vi "ma_SML Averaged FFT Power Spectrum.vi"(6 "reset averaging?":bool, 8 "error in (no error)":errorcluster, 9 "averaging parameters":T1={"averaging type"=enum."no averaging", "averaging settings"={"weighting type"=enum."linear", "weighting settings"={"size"=10.0, "linear weighting mode"=enum."moving average"}}}, 10 "spectral info in":T5 {"window" items=["Rectangle"=0, "Hanning"=1, "Hamming"=2, "Blackman-Harris"=3, "Exact Blackman"=4, "Blackman"=5, "Flat Top"=6, "4 Term B-Harris "=7, "7 Term B-Harris"=8, "Low Sidelobe"=9, "Blackman Nuttall"=11, "Triangle"=30, "Bartlett-Hanning"=31, "Bohman"=32, "Parzen"=33, "Welch"=34, "Kaiser"=60, "Dolph-Chebyshev"=61, "Gaussian"=62]}, 11 "FFT spectrum":T4 {"spectrum" format="%.2f"; "df" format="%.2f"; "f0" format="%.2f"}) -> (0 "error out":errorcluster, 1 "data ready?":bool, 2 "spectral info out":T5 {"window" items=["Rectangle"=0, "Hanning"=1, "Hamming"=2, "Blackman-Harris"=3, "Exact Blackman"=4, "Blackman"=5, "Flat Top"=6, "4 Term B-Harris "=7, "7 Term B-Harris"=8, "Low Sidelobe"=9, "Blackman Nuttall"=11, "Triangle"=30, "Bartlett-Hanning"=31, "Bohman"=32, "Parzen"=33, "Welch"=34, "Kaiser"=60, "Dolph-Chebyshev"=61, "Gaussian"=62]}, 3 "avg power spectrum":T3 {"spectrum" format="%.2f"; "df" format="%.2f"; "f0" format="%.2f"}, 4 "averages sofar":dbl)   [LabVIEW 2020, in "NI_MAPro.lvlib"]
uses:
  NI_MAPro.lvlib
  ma_sml_Spectral Info.ctl
  ma_sml_Spectrum Cluster (complex).ctl
  ma_sml_Spectrum Cluster (real).ctl
  ma_sml_Averaging Parameters.ctl
  ma_sml_Averaging Settings.ctl
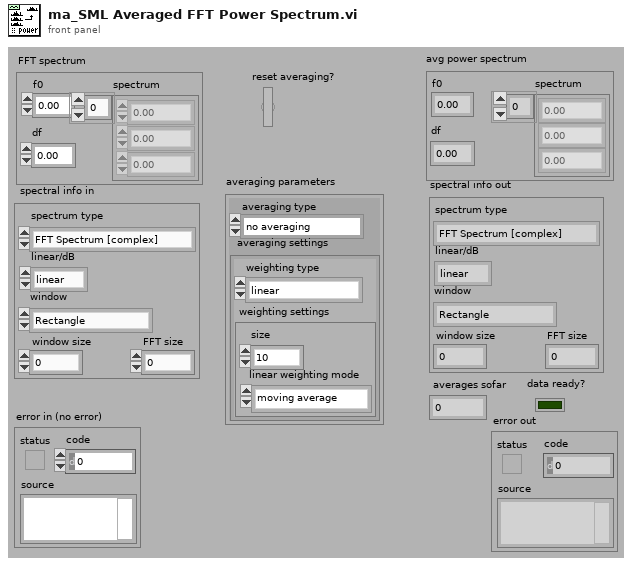
[diagram p1: front panel]
types:
  T1 = typedef "NI_MAPro.lvlib/ma_sml_Averaging Parameters.ctl" = cluster{"averaging type":enum16{"no averaging", "vector averaging", "RMS averaging", "peak hold"}, "averaging settings":T2}
  T2 = typedef "NI_MAPro.lvlib/ma_sml_Averaging Settings.ctl" = cluster{"weighting type":enum16{"linear", "exponential"}, "weighting settings":cluster{"size":dbl, "linear weighting mode":enum16{"one shot", "auto restart one shot", "moving average", "continuous"}}}
  T3 = typedef "NI_MAPro.lvlib/ma_sml_Spectrum Cluster (real).ctl" = cluster{"f0":dbl, "df":dbl, "spectrum":dbl[]}
  T4 = typedef "NI_MAPro.lvlib/ma_sml_Spectrum Cluster (complex).ctl" = cluster{"f0":dbl, "df":dbl, "spectrum":cdb[]}
  T5 = typedef "NI_MAPro.lvlib/ma_sml_Spectral Info.ctl" = cluster{"spectrum type":enum16{"FFT Spectrum [complex]", "Amplitude [Magnitude]", "Power [Magnitude^2]", "Cross Spectrum [complex]", "Frequency Response [Complex]"}, "linear/dB":enum16{"linear", "dB"}, "window":u16, "window size":i32, "FFT size":i32}
  T6 = enum16{"FFT Spectrum [complex]", "Amplitude [Magnitude]", "Power [Magnitude^2]", "Cross Spectrum [complex]", "Frequency Response [Complex]"}
  T7 = enum16{"no averaging", "vector averaging", "RMS averaging", "peak hold"}
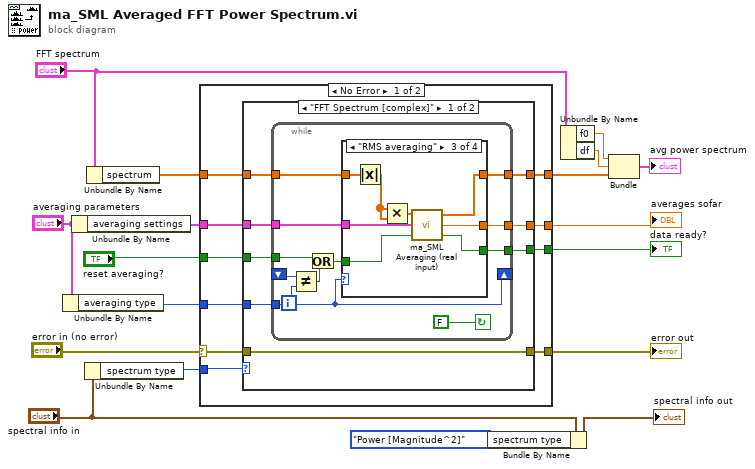
[diagram p0: block diagram]
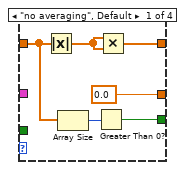
[diagram p2: hidden frame]
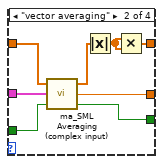
[diagram p3: hidden frame]
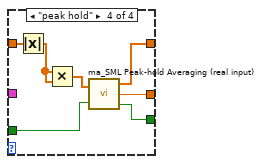
[diagram p4: hidden frame]
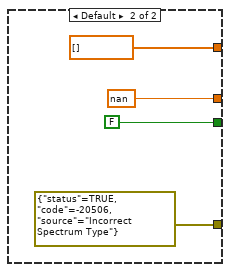
[diagram p5: hidden frame]
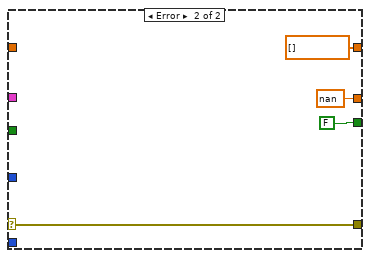
[diagram p6: hidden frame]
diagram:
  n1 = Unbundle By Name("averaging parameters") -> ("averaging type"=w7:T7)
  n2 = Unbundle By Name("averaging parameters") -> ("averaging settings"=w9:T2)
  n3 = Unbundle By Name("spectral info in") -> ("spectrum type"=w12:T6)
  n4 = Unbundle By Name("FFT spectrum") -> ("spectrum"=w16:cdb[])
  n5 = case shown="No Error" "error in (no error)" {
    selector: "error in (no error)" -> [w19 w81]
    tunnel: [w22 FALSE ("Data Ready")] -> w18
    tunnel: [w28 nan ("Averaged So-far")] -> w17
    tunnel: [w27 dbl[] [] ("y")] -> w14
    tunnel: w7 -> [w26 _]
    tunnel: w9 -> [w25 _]
    tunnel: "reset averaging?" -> [w24 _]
    tunnel: w16 -> [w23 _]
    tunnel: [w20 w81] -> w3
    tunnel: w12 -> [w21 _]
    frame No Error {
      n6 = case shown="\"FFT Spectrum [complex]\"" w21 {
        tunnel: [w36 nan ("Averaged So-far")] -> w28
        tunnel: [w35 dbl[] [] ("y")] -> w27
        tunnel: w26 -> [w34 _]
        tunnel: w25 -> [w33 _]
        tunnel: w24 -> [w32 _]
        tunnel: w23 -> [w29 _]
        tunnel: [w30 FALSE] -> w22
        tunnel: w19 -> [w31 _]
        tunnel: [w31 errorcluster {"status"=TRUE, "code"=-20506, "source"="Incorrect Spectrum Type"} ("error in (no error)")] -> w20
        frame "FFT Spectrum [complex]" {
          n7 = while {
            tunnel: w33 -> [w40]
            shift-left: _ -> [w38]
            shift-right: [w37] -> _
            tunnel: w34 -> [w37]
            tunnel: w32 -> [w42]
            tunnel: [w44] -> w36
            tunnel: [w45] -> w30
            tunnel: [w46] -> w35
            tunnel: w29 -> [w47]
            stop <- FALSE continue-if-true
            n8 = Not Equal?(x=w38, y=w37) -> (x != y?=w41:bool)
            n9 = Or(x=w42, y=w41) -> (x .or. y?=w43:bool)
            n10 = case shown="\"RMS averaging\"" w37 {
              tunnel: [w52 w56 w63 w74] -> w46
              tunnel: w47 -> [w50 w61 w69 w75]
              tunnel: [w48 w58 w65 w70] -> w45
              tunnel: [0.0 ("Averaged So-far") w59 w66 w73] -> w44
              tunnel: w43 -> [_ w60 w64 w76]
              tunnel: w40 -> [_ w54 w62 _]
              frame "no averaging", Default {
                n11 = Absolute Value(x=w50) -> (abs(x)=w51:dbl[])
                n12 = Array Size(array=w50) -> (size(s)=w49:i32)
                n13 = Greater Than 0?(x=w49) -> (x > 0?=w48:bool)
                n14 = Multiply(x=w51, y=w51) -> (x*y=w52:dbl[])
              }
              frame "vector averaging" {
                n15 = call "ma_SML Averaging (complex input).vi"("reset?"=w60, "averaging settings"=w54, "x"=w61) -> ("data ready?"=w58:bool, "averaged sofar"=w59:dbl, "y"=w57:cdb[])
                n16 = Absolute Value(x=w57) -> (abs(x)=w55:dbl[])
                n17 = Multiply(x=w55, y=w55) -> (x*y=w56:dbl[])
              }
              frame "RMS averaging" {
                n18 = Absolute Value(x=w69) -> (abs(x)=w67:dbl[])
                n19 = Multiply(x=w67, y=w67) -> (x*y=w68:dbl[])
                n20 = call "ma_SML Averaging (real input).vi"("reset?"=w64, "averaging settings"=w62, "x"=w68) -> ("data ready?"=w65:bool, "averaged sofar"=w66:dbl, "y"=w63:dbl[])
              }
              frame "peak hold" {
                n21 = Absolute Value(x=w75) -> (abs(x)=w71:dbl[])
                n22 = Multiply(x=w71, y=w71) -> (x*y=w72:dbl[])
                n23 = call "ma_SML Peak-hold Averaging (real input).vi"("x"=w72, "reset?"=w76) -> ("y"=w74:dbl[], "averages sofar"=w73:dbl, "data ready?"=w70:bool)
              }
            }
          }
        }
        frame Default {
        }
      }
    }
    frame Error {
    }
  }
  "error out" <- w3
  "data ready?" <- w18
  "averages sofar" <- w17
  n24 = Bundle By Name(cluster="spectral info in", "spectrum type"=T6."Power [Magnitude^2]") -> (→"spectral info out":T5)
  n25 = Unbundle By Name("FFT spectrum") -> ("f0"=w6:dbl, "df"=w5:dbl)
  n26 = Bundle("f0"=w6, "df"=w5, "y"=w14) -> (→"avg power spectrum":cluster{"f0":dbl, "df":dbl, "y":dbl[]})  [unwired: 1 out]
